vi "Main Interface.vi"() -> ()   [LabVIEW 2015]
uses:
  FPGA/Rate.ctl
  Reusable/CRDS/Data/Cell/extparam.ctl
  Devices/Alicat/Session Based/Data/M/M data.lvclass
  <vilib>/Utility/miscctls.llb/LVPositionTypeDef.ctl
  CRD/Data/tCRD Data.lvclass
  CRD/Data/tCRD Data.lvclass/tCRD Data.ctl
  Reusable/CRDS/Data/Cell/CRDS Cell Data.lvclass/CRDS Cell Data.ctl
  <vilib>/event_ctls.llb/eventvkey.ctl
  CRD/Data/Accessors/Read file path.vi
  CRD/Data/Accessors/Read file size.vi
  Reusable/CRDS/Data/Cell/Read extParam.vi
  Reusable/CRDS/Data/Cell/Read FitCoeff.vi
  Reusable/Data/Read measTime.vi
  Reusable/CRDS/Data/Main/Read CellData.vi
  Reusable/CRDS/Data/Cell/Read Ringdowns.vi
  <vilib>/Analysis/1siggen.llb/Ramp Pattern by Delta.vi
  Reusable/CRDS/Data/Cell/CRDS Cell Data.lvclass
  Reusable/General/Math Utilities.lvlib
  <vilib>/Analysis/NI_AALBase.lvlib
panel:
  in  "writeTaus":bool
  in  "newFile":bool
  in  "restart":bool
  in  "SyncTime":bool
  in  "writeRDs":bool
  in  "mainTab":enum32{"Main", "Control"}(tab)
  out "rd":dbl[][](graph)
  out "tau (us)":sgl
  out "Data In":sgl(graph)
  out "eRD":dbl[](graph)
  in  "Invert?":bool
  out "Drive Space (Mb)":u32
  in  "Laser Off (us)":u32=16
  in  "# to Coadd":u8=16 min=1 max=50 step=1
  in  "Rate":T1=10 items=["1 MHz"=20, "2 MHz"=10, "2.5 MHz"=8, "5 MHz"=4, "10 MHz"=2, "20MHz"=1]
  in  "Sample Time (us)":u16=100
  in  "Delay (us)":u16=16
  in  "Frequency (Hz)":dbl
  out "Path":path
  out "File Size":u32
  out "extParam":T2={"Tau"=nan, "Tau0cor"=nan, "ext"=nan, "extCorr"=nan, "stdevTau"=nan, "eTau"=nan, "taucorr"=nan, "Tau0"=nan, "max"=nan} caption="Extinction Parameters" {"Tau0" format="%#.2f"; "taucorr" format="%#.2f"; "eTau" format="%#.2f"; "stdevTau" format="%#.2f"; "extCorr" format="%.2f"; "ext" format="%#.2f"; "Tau0cor" format="%#.2f"; "Tau" format="%#.2f"}
  out "Version":string
  in  "Save":bool
  out "time":timestamp format="%<%H:%M:%S%2u>T"
  # "OPEN PATH DATA"
  # "CONTROL"
  # "Open Path CRD Control"
  # "Laser/Sample Control"
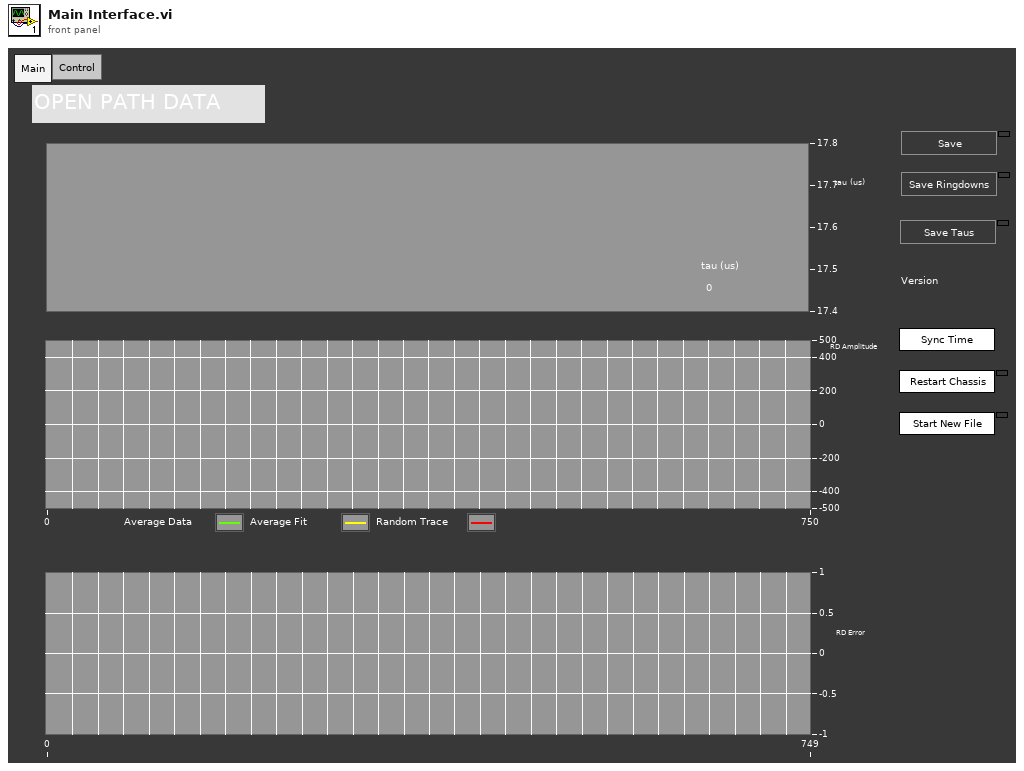
[diagram p1: front panel]
types:
  T1 = typedef "Rate.ctl" = u8
  T2 = typedef "extparam.ctl" = cluster{"Tau":sgl, "Tau0cor":sgl, "ext":sgl, "extCorr":sgl, "stdevTau":sgl, "eTau":sgl, "taucorr":sgl, "Tau0":sgl, "max":sgl}
  T3 = enum32{"Invalid", "Standard", "Closed", "Hidden", "Minimized", "Maximized"}
  T4 = typedef "LVPositionTypeDef.ctl" = cluster{"Left":i32, "Top":i32}
  T5 = typedef "eventvkey.ctl" = enum16{"ASCII", "Enter", "Return", "Shift", "Ctrl", "Alt", "Cmd", "Opt", "Caps", "NumLock", "Clear", "Break", "Up", "Down", "Left", "Right", "Insert", "Delete", "Home", "End", "PageUp", "PageDown", "Escape", "Help", "Pause", "ScrollLock", "F1", "F2", "F3", "F4", "F5", "F6", "F7", "F8", "F9", "F10", "F11", "F12", "F13", "F14", "F15", "F16", "F17", "F18", "F19", "F20", "F21", "F22", "F23", "F24", "Play", "VolumeUp", "VolumeDown", "Mute", "Two Byte Char"}
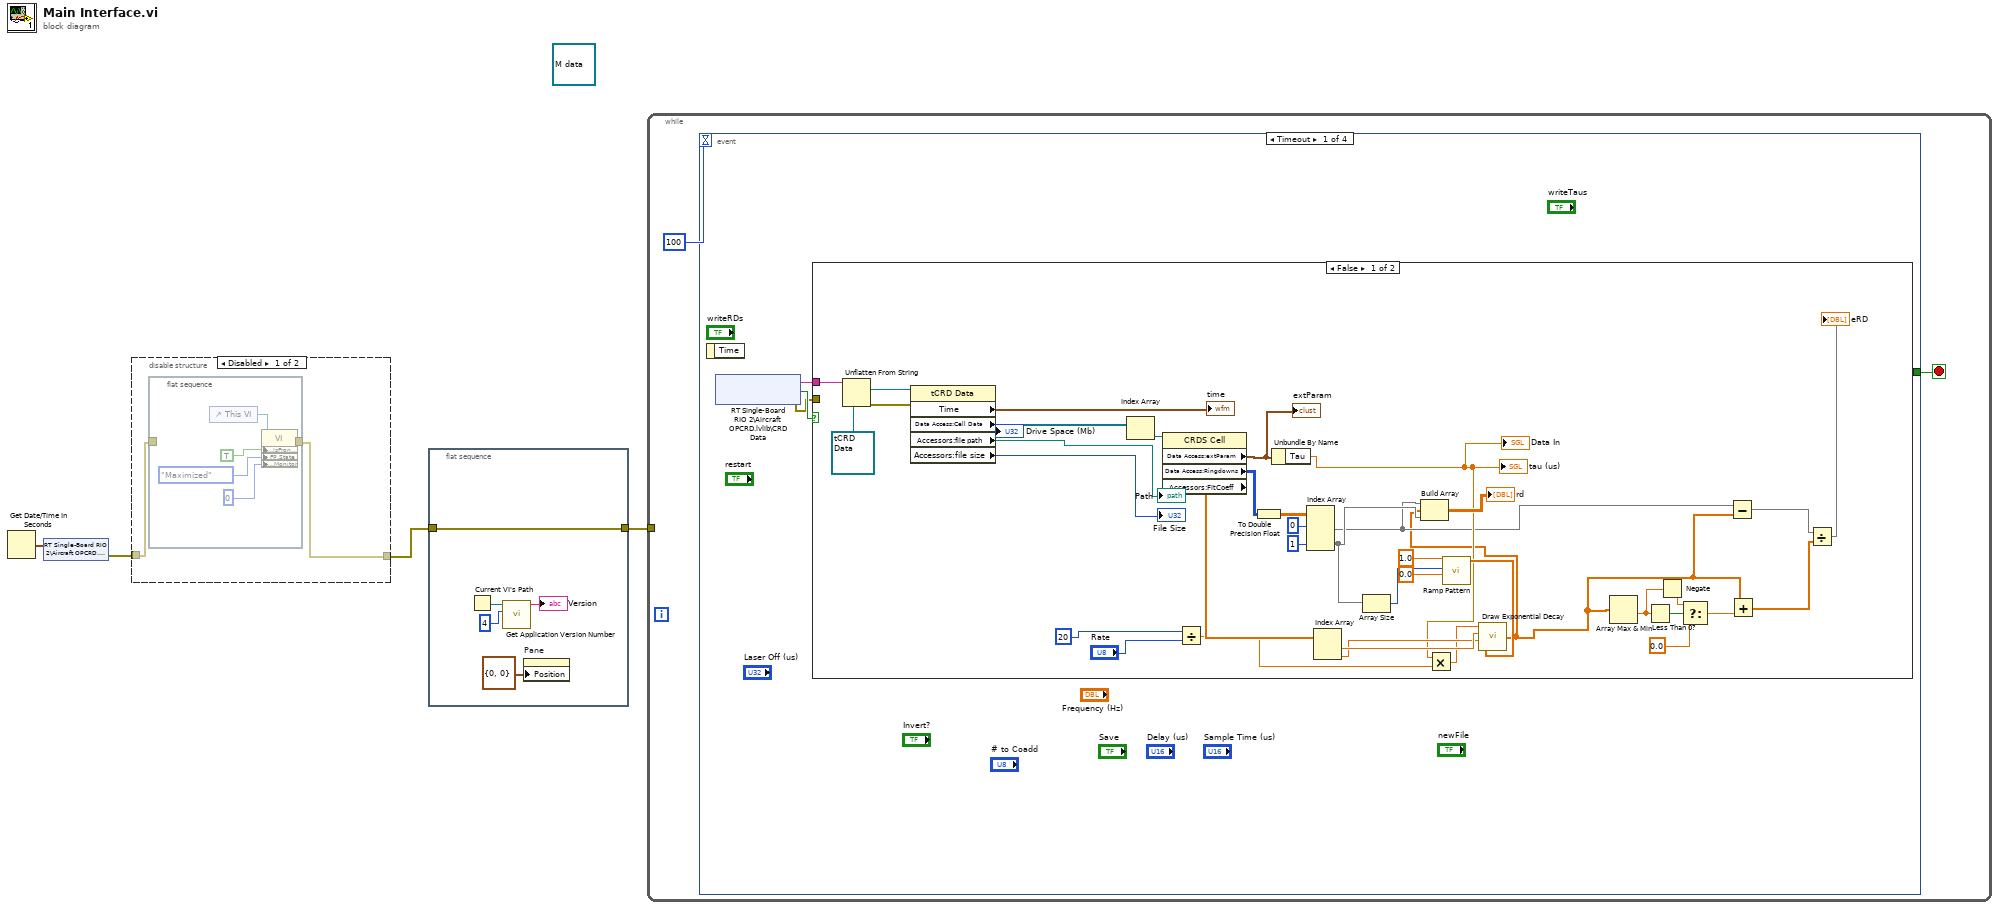
[diagram p0: block diagram]
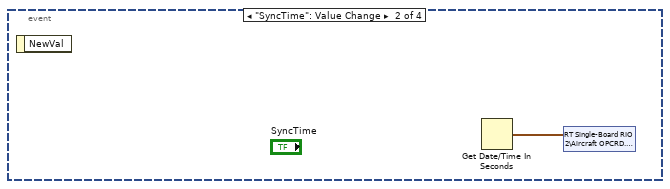
[diagram p4: hidden frame]
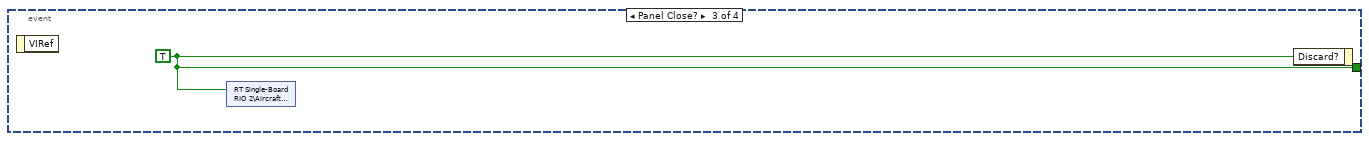
[diagram p5: hidden frame]
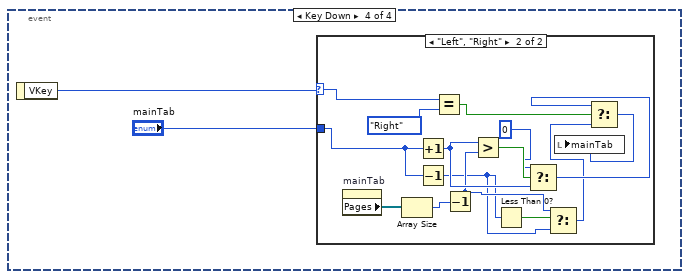
[diagram p6: hidden frame]
diagram:
  (unwired) refnum<class "M data.lvclass"> refnum ("M Data")
  n1 = Get Date/Time In Seconds() -> (seconds since 1Jan1904=w4:timestamp)
  n2 = shared-variable "RT Single-Board RIO 2\\Aircraft OPCRD.lvlib\\Time"(w4) -> (error out=w3:errorcluster)  [unwired: 1 in]
  n3 = disable-structure shown="Disabled" {
    disable-tunnel: w3 -> [w6 w12]
    disable-tunnel: [w5 w12] -> w2
    frame Disabled {
      n4 = flat-sequence {
        tunnel: [w7] -> w5
        tunnel: w6 -> [_]
        frame #0 {
          n5 = control-ref of="This VI"() -> (w11:refnum<vi>)
          n6 = property class="VI"(reference=w11, "Front Panel.IsFrontmost"=TRUE ("Front Panel Window:Is Frontmost"), "FP.State"=T3."Maximized" ("Front Panel Window:State"), "FP.Monitor"=u16 0 ("Front Panel Window:Monitor")) -> (error out=w7:errorcluster)  [unwired: 1 in, 1 out]
        }
      }
    }
    frame Enabled {
    }
  }
  n7 = flat-sequence {
    tunnel: w2 -> [w13]
    tunnel: [w13] -> w1
    frame #0 {
      n8 = Current VI's Path() -> (path=w15:path)
      n9 = call "Get Application Version Number.vi"("Number to Strip"=4, "Initial Path"=w15) -> ("Version"=→"Version":string)  [unwired: 8 in, 1 out]
      n10 = property on="Pane" class="Pane"("Position"=T4 {"Left"=0, "Top"=0}) -> ()  [unwired: 2 in, 2 out]
    }
  }
  n11 = while {
    tunnel: w1 -> [_]
    stop <- w19 stop-if-true
    n12 = event shown="[0] Timeout" {
      selector: _ -> [_ _ _ _]
      dyn-events: _ -> [_ _ _ _]
      timeout: 100 -> [_ _ _ _]
      tunnel: [_ _ w62 _] -> w19
      event Timeout {
        n13 = event-data() -> ()  [unwired: 1 in, 1 out]
        n14 = shared-variable "RT Single-Board RIO 2\\Aircraft OPCRD.lvlib\\CRD Data"() -> (w22:string, error out=w20:errorcluster, w21:bool)  [unwired: 2 in]
        n15 = case shown="False" w21 {
          tunnel: w22 -> [w60 _]
          tunnel: w20 -> [_ _]
          frame False {
            n16 = Unflatten From String(type=refnum<class "tCRD Data.lvclass"> refnum ("tCRD Data"), binary string=w60) -> (value=w59:refnum<class "tCRD Data.lvclass">, error out=w58:errorcluster)  [unwired: 3 in, 1 out]
            n17 = property class="tCRD Data"(reference=w59, error in=w58) -> ("Time"=→"time":timestamp, "Data Access:Cell Data"=w57:refnum<class "CRDS Cell Data.lvclass">[], "Accessors:file path"=→"Path":path, "Accessors:file size"=→"File Size":u32)  [unwired: 2 out]
            n18 = Index Array(array=w57) -> (element=w56:refnum<class "CRDS Cell Data.lvclass">)  [unwired: 1 in]
            n19 = property class="CRDS Cell"(reference=w56) -> ("Data Access:extParam"=w47:T2, "Data Access:Ringdowns"=w50:i16[][], "Accessors:FitCoeff"=w46:dbl[])  [unwired: 1 in, 2 out]
            "extParam" <- w47
            n20 = Divide(x=20, y="Rate") -> (x/y=w34:dbl)
            n21 = To Double Precision Float(number=w50) -> (double precision float=w49:dbl[][])
            n22 = Unbundle By Name(w47) -> ("Tau"=w35:sgl)
            "Data In" <- w35
            "tau (us)" <- w35
            n23 = Index Array(array=w49, index (row) #1=0 ("index (row)"), index (row) #2=1 ("index (row)")) -> (element #1=w27:dbl[], element #2=w41:dbl[])  [unwired: 2 in]
            n24 = Index Array(array=w46) -> (element #1=w45:dbl, element #2=w44:dbl)  [unwired: 2 in]
            n25 = Array Size(array=w41) -> (size(s)=w40:i32)
            n26 = Multiply(x=w35, y=w34) -> (x*y=w33:dbl)
            n27 = call-poly <vilib>:"Ramp Pattern.vi"("start"=0.0, "end"=w40, "delta"=1.0) -> ("Ramp Pattern"=w43:dbl[])  [unwired: 6 in, 2 out]
            n28 = call "Draw Exponential Decay.vi"("time"=w43, "B"=w44, "A"=w45, "tau"=w33) -> ("ExponentialOut"=w23:dbl[])
            n29 = Build Array(w27, w23, w41) -> (→"rd":dbl[][])
            n30 = Array Max & Min(array=w23) -> (min value=w25:dbl)  [unwired: 3 out]
            n31 = Less Than 0?(x=w25) -> (x < 0?=w32:bool)
            n32 = Negate(x=w25) -> (-x=w24:dbl)
            n33 = Select(t=w24, s=w32, f=0.0) -> (s? t:f=w26:dbl)
            n34 = Subtract(x=w27, y=w23) -> (x-y=w30:dbl[])
            n35 = Add(x=w23, y=w26) -> (x+y=w28:dbl[])
            n36 = Divide(x=w30, y=w28) -> (x/y=→"eRD":dbl[])
          }
          frame True {
          }
        }
      }
      event "SyncTime": Value Change {
        n37 = event-data() -> ()  [unwired: 1 in, 1 out]
        n38 = Get Date/Time In Seconds() -> (seconds since 1Jan1904=w61:timestamp)
        n39 = shared-variable "RT Single-Board RIO 2\\Aircraft OPCRD.lvlib\\Time"(w61) -> ()  [unwired: 1 in, 1 out]
      }
      event Panel Close? {
        w62 = TRUE ("Discard?")
        n40 = event-data() -> ()  [unwired: 1 in, 1 out]
        n41 = shared-variable "RT Single-Board RIO 2\\Aircraft OPCRD.lvlib\\Stop"(w62) -> ()  [unwired: 1 in, 1 out]
        n42 = event-data("Discard?"=w62) -> ()  [unwired: 1 in, 1 out]
      }
      event Key Down {
        n43 = event-data() -> ("VKey"=w64:T5)  [unwired: 1 in]
        n44 = case shown="\"Left\", \"Right\"" w64 {
          selector: w64 -> [_ w78]
          tunnel: "mainTab" -> [_ w70]
          frame "ASCII", Default {
          }
          frame "Left", "Right" {
            n45 = property on="mainTab" class="TabCtl (strict)"() -> ("Pages"=w79:refnum<vi>[])  [unwired: 2 in, 2 out]
            n46 = Array Size(array=w79) -> (size(s)=w75:i32)
            n47 = Increment(x=w70) -> (x+1=w73:enum32{"Main", "Control"})
            n48 = Decrement(x=w70) -> (x-1=w67:enum32{"Main", "Control"})
            n49 = Equal?(x=w78, y=eventvkey."Right") -> (x = y?=w76:bool)
            n50 = Decrement(x=w75) -> (x-1=w68:i32)
            n51 = Greater?(x=w73, y=w68) -> (0:w74:bool)
            n52 = Less Than 0?(x=w67) -> (x < 0?=w69:bool)
            n53 = Select(t=0, s=w74, f=w73) -> (s? t:f=w71:u32)
            n54 = Select(t=w68, s=w69, f=w67) -> (s? t:f=w66:u32)
            n55 = Select(t=w71, s=w76, f=w66) -> (s? t:f=w65:u32)
            n56 = local write "mainTab"(w65) -> ()
          }
        }
      }
    }
  }
